vi "create complex region.vi"(7 "scale factor":dbl=1.0, 11 "z in window":cdb[](array[numeric])) -> (3 "complex region":T1)   [LabVIEW 2010]
uses:
  complex region.ctl
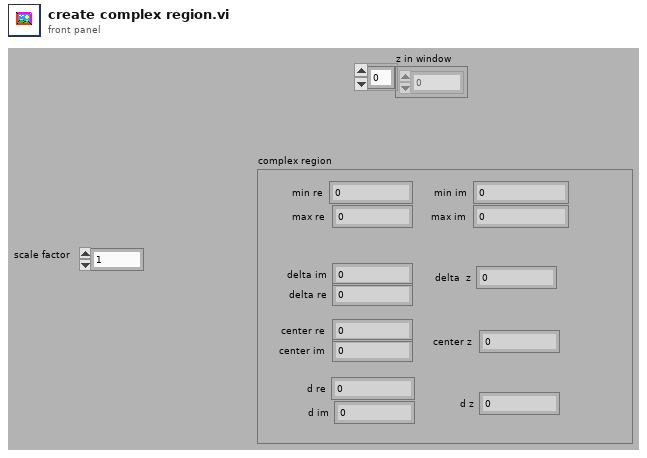
[diagram p1: front panel]
types:
  T1 = typedef "complex region.ctl" = cluster{"max re":dbl, "min re":dbl, "max im":dbl, "min im":dbl, "delta re":dbl, "delta im":dbl, "center re":dbl, "delta  z":cdb, "center im":dbl, "center z":cdb, "d im":dbl, "d re":dbl, "d z":cdb}
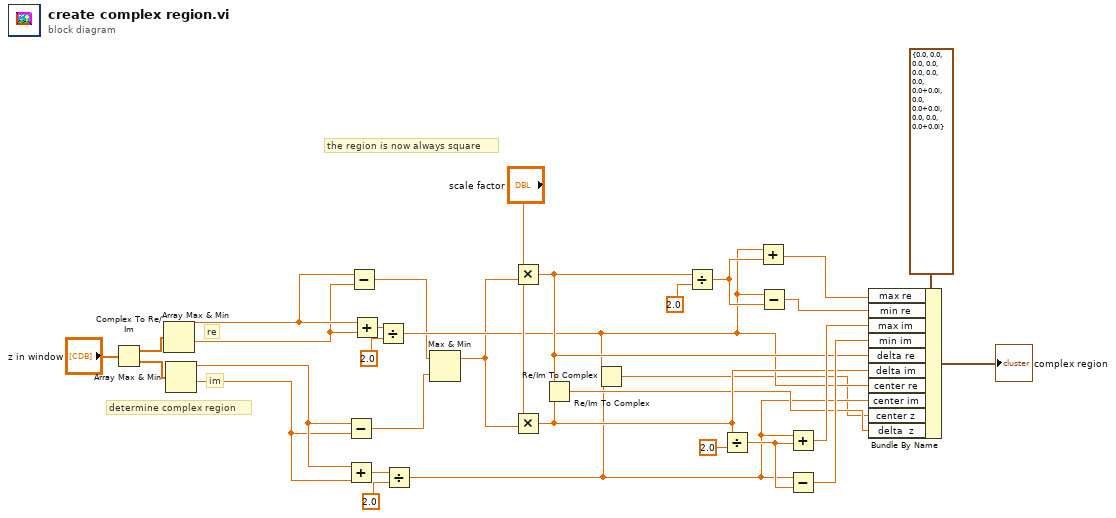
[diagram p0: block diagram]
diagram:
  # "the region is now always square"
  # "determine complex region"
  # "im"
  # "re"
  n1 = Complex To Re/Im(x + iy="z in window") -> (x=w18:dbl[], y=w17:dbl[])
  n2 = Array Max & Min(array=w18) -> (max value=w12:dbl, min value=w11:dbl)  [unwired: 2 out]
  n3 = Array Max & Min(array=w17) -> (max value=w15:dbl, min value=w14:dbl)  [unwired: 2 out]
  n4 = Subtract(x=w15, y=w14) -> (x-y=w2:dbl)
  n5 = Add(x=w15, y=w14) -> (x+y=w13:dbl)
  n6 = Subtract(x=w12, y=w11) -> (x-y=w3:dbl)
  n7 = Add(x=w12, y=w11) -> (x+y=w10:dbl)
  n8 = Divide(x=w10, y=2.0) -> (x/y=w6:dbl)
  n9 = Divide(x=w13, y=2.0) -> (x/y=w5:dbl)
  n10 = Max & Min(x=w3, y=w2) -> (max(x,y)=w1:dbl)  [unwired: 1 out]
  n11 = Multiply(x="scale factor", y=w1) -> (x*y=w9:dbl)
  n12 = Multiply(x="scale factor", y=w1) -> (x*y=w8:dbl)
  n13 = Re/Im To Complex(1:w8, 2:w9) -> (0:w7:cdb)
  n14 = Re/Im To Complex(1:w5, 2:w6) -> (0:w4:cdb)
  n15 = Divide(x=w9, y=2.0) -> (x/y=w24:dbl)
  n16 = Divide(x=w8, y=2.0) -> (x/y=w21:dbl)
  n17 = Add(x=w6, y=w24) -> (x+y=w25:dbl)
  n18 = Subtract(x=w6, y=w24) -> (x-y=w23:dbl)
  n19 = Add(x=w5, y=w21) -> (x+y=w20:dbl)
  n20 = Subtract(x=w5, y=w21) -> (x-y=w19:dbl)
  n21 = Bundle By Name(cluster=T1 {"max re"=0.0, "min re"=0.0, "max im"=0.0, "min im"=0.0, "delta re"=0.0, "delta im"=0.0, "center re"=0.0, "delta  z"=0.0+0.0i, "center im"=0.0, "center z"=0.0+0.0i, "d im"=0.0, "d re"=0.0, "d z"=0.0+0.0i} ("complex region"), "max re"=w25, "min re"=w23, "max im"=w20, "min im"=w19, "delta re"=w9, "delta im"=w8, "center re"=w6, "center im"=w5, "center z"=w4, "delta  z"=w7) -> (→"complex region":T1)
